vi "trlbase.vi"() -> ()   [LabVIEW 2021]
panel:
  in  "stop":bool
  out "TL 4":cluster{"Green":bool, "Amber":bool, "Red":bool}
  out "TL 3":cluster{"Green":bool, "Amber":bool, "Red":bool}
  out "TL 2":cluster{"Green":bool, "Amber":bool, "Red":bool}
  out "TL1":cluster{"Green":bool, "Amber":bool, "Red":bool}
  in  "Ped1":bool
  in  "Ped 2":bool
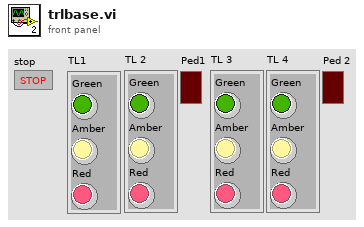
[diagram p1: front panel]
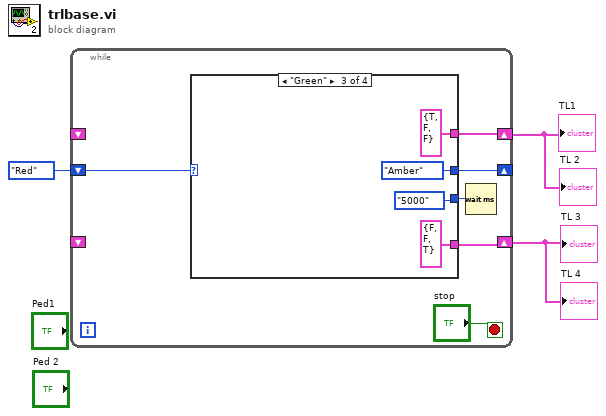
[diagram p0: block diagram]
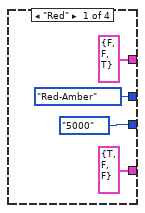
[diagram p2: hidden frame]
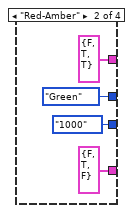
[diagram p3: hidden frame]
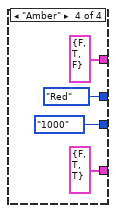
[diagram p4: hidden frame]
diagram:
  n1 = while {
    shift-right: [w9] -> _
    shift-left: enum16{"Amber", "Green", "Red-Amber", "Red"}."Red" ("Enum") -> [w8]
    shift-right: [w4] -> w1
    shift-left: _ -> [_]
    shift-right: [w5] -> w2
    shift-left: _ -> [_]
    stop <- "stop" stop-if-true
    n2 = case shown="\"Green\"" w8 {
      tunnel: [cluster{"Green":bool, "Amber":bool, "Red":bool} {"Green"=FALSE, "Amber"=FALSE, "Red"=TRUE} ("TL1") cluster{"Green":bool, "Amber":bool, "Red":bool} {"Green"=FALSE, "Amber"=TRUE, "Red"=TRUE} ("TL1") cluster{"Green":bool, "Amber":bool, "Red":bool} {"Green"=TRUE, "Amber"=FALSE, "Red"=FALSE} ("TL1") cluster{"Green":bool, "Amber":bool, "Red":bool} {"Green"=FALSE, "Amber"=TRUE, "Red"=FALSE} ("TL1")] -> w4
      tunnel: [cluster{"Green":bool, "Amber":bool, "Red":bool} {"Green"=TRUE, "Amber"=FALSE, "Red"=FALSE} ("TL1") cluster{"Green":bool, "Amber":bool, "Red":bool} {"Green"=FALSE, "Amber"=TRUE, "Red"=FALSE} ("TL1") cluster{"Green":bool, "Amber":bool, "Red":bool} {"Green"=FALSE, "Amber"=FALSE, "Red"=TRUE} ("TL1") cluster{"Green":bool, "Amber":bool, "Red":bool} {"Green"=FALSE, "Amber"=TRUE, "Red"=TRUE} ("TL1")] -> w5
      tunnel: [enum16{"Amber", "Green", "Red-Amber", "Red"}."Red-Amber" ("Enum") enum16{"Amber", "Green", "Red-Amber", "Red"}."Green" ("Enum") enum16{"Amber", "Green", "Red-Amber", "Red"}."Amber" ("Enum") enum16{"Amber", "Green", "Red-Amber", "Red"}."Red" ("Enum")] -> w9
      tunnel: [enum16{"5000"}."5000" enum16{"1000"}."1000" enum16{"5000"}."5000" enum16{"1000"}."1000"] -> w6
      frame "Red" {
      }
      frame "Red-Amber" {
      }
      frame "Green" {
      }
      frame "Amber" {
      }
    }
    n3 = Wait (ms)(milliseconds to wait=w6) -> ()  [unwired: 1 out]
  }
  "TL1" <- w1
  "TL 2" <- w1
  "TL 3" <- w2
  "TL 4" <- w2
